vi "Find Roughness and Standard Deviation.vi"(9 "Standard Deviation":refnum<queue>, 10 "History Average":refnum<queue>, 11 "Video Frame in":refnum<class "Video Frame.lvclass">) -> (2 "elements":dbl[](array[numeric]), 3 "Column Averages":dbl[](array[numeric]))   [LabVIEW 2018]
uses:
  Classes/Video Frame/Video Frame.lvclass
  <vilib>/Analysis/NI_AALBase.lvlib
  b6131b5e-4e8b-4e5f-a1e4-30dca00ce91b.vi
  0d0c4324-7153-4ce5-a3f6-87b0ea44ce7f.vi
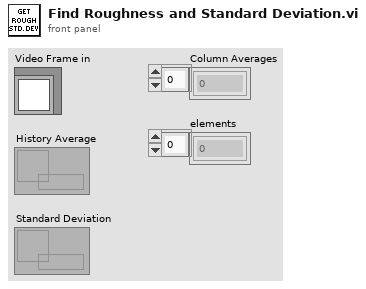
[diagram p1: front panel]
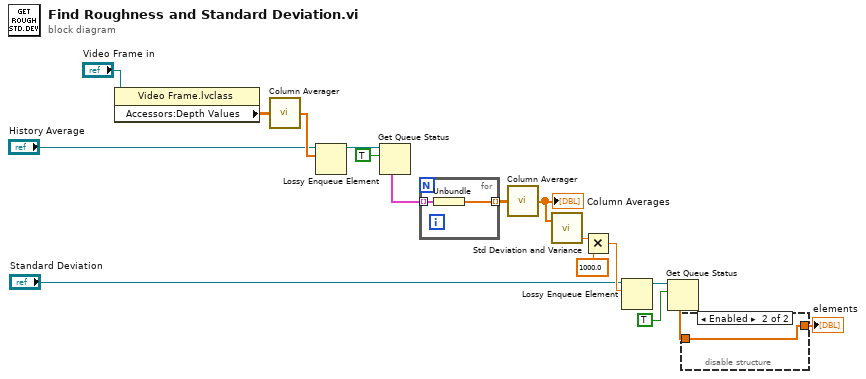
[diagram p0: block diagram]
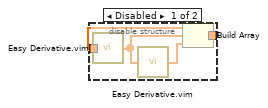
[diagram p2: hidden frame]
diagram:
  n1 = property class="Video Frame.lvclass"(reference="Video Frame in") -> ("Accessors:Depth Values"=w2:dbl[][])  [unwired: 1 in, 2 out]
  n2 = call "Column Averager.vi"("Depth Values"=w2) -> ("Column Averages"=w4:dbl[])
  n3 = Lossy Enqueue Element(queue="History Average", element=w4) -> (queue out=w5:refnum<queue>)  [unwired: 1 in, 3 out]
  n4 = Get Queue Status(queue=w5, return elements? (F)=TRUE) -> (elements=w7:cluster{dbl[]}[])  [unwired: 1 in, 7 out]
  n5 = for {
    tunnel: w7 -> [w19] mode=indexing
    tunnel: [w18] -> w8 mode=indexing
    n6 = Unbundle(w19) -> (w18:dbl[])
  }
  n7 = call "Column Averager.vi"("Depth Values"=w8) -> ("Column Averages"=w9:dbl[])
  "Column Averages" <- w9
  n8 = call <vilib>:"Std Deviation and Variance.vi"("X"=w9) -> ("variance"=w10:dbl)  [unwired: 1 in, 2 out]
  n9 = Multiply(x=w10, y=1000.0) -> (x*y=w13:dbl)
  n10 = Lossy Enqueue Element(queue="Standard Deviation", element=w13) -> (queue out=w14:refnum<queue>)  [unwired: 1 in, 3 out]
  n11 = Get Queue Status(queue=w14, return elements? (F)=TRUE) -> (elements=w16:dbl[])  [unwired: 1 in, 7 out]
  n12 = disable-structure shown="Enabled" {
    disable-tunnel: [w23 w24] -> w15
    disable-tunnel: w16 -> [w22 w24]
    frame Disabled {
      n13 = call "Easy Derivative.vim"("X"=w22) -> ("dX/dt"=w21:dbl[])  [unwired: 14 in]
      n14 = call "Easy Derivative.vim"("X"=w21) -> ("dX/dt"=w20:dbl[])  [unwired: 14 in]
      n15 = Build Array(w22, w21, w20) -> (w23:dbl[][])
    }
    frame Enabled {
    }
  }
  "elements" <- w15
